vi "get control size.vi"(8 "error in (no error)":errorcluster, 11 "Control in":refnum<class "String Control.lvclass">) -> (0 "error out":errorcluster, 2 "Size":T1, 3 "Control out":refnum<class "String Control.lvclass">)   [LabVIEW 2010, in "String Control.lvclass"]
uses:
  String Control.lvclass
  <vilib>/Utility/miscctls.llb/LVBoundsTypeDef.ctl
  String Control.lvclass/String Control.ctl
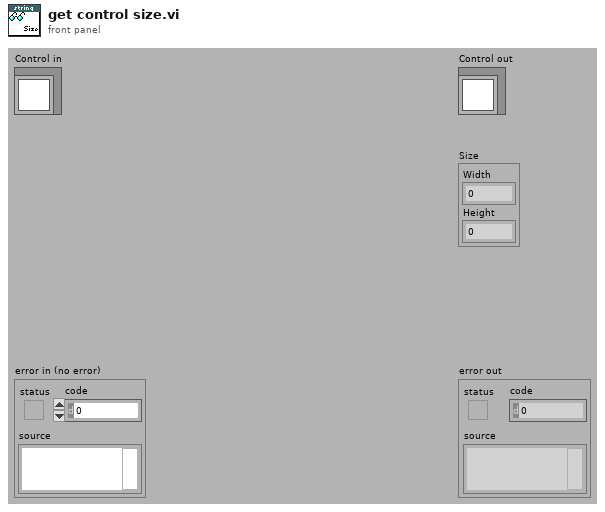
[diagram p1: front panel]
types:
  T1 = typedef "LVBoundsTypeDef.ctl" = cluster{"Width":u32, "Height":u32}
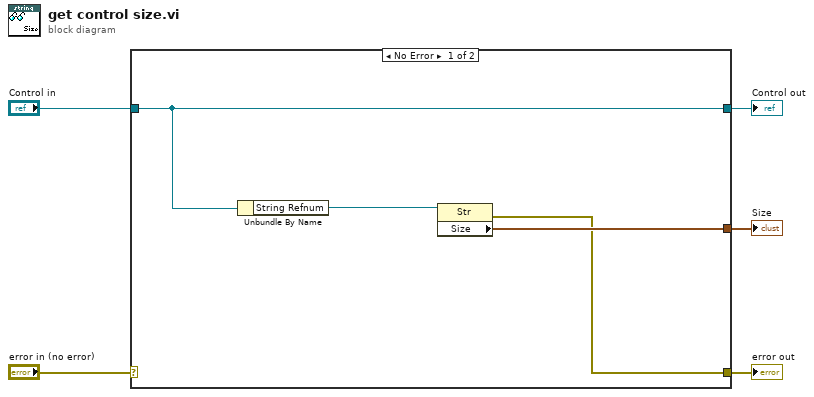
[diagram p0: block diagram]
diagram:
  n1 = case shown="No Error" "error in (no error)" {
    selector: "error in (no error)" -> [_ w11]
    tunnel: [w8 w11] -> w4
    tunnel: [w7 w10] -> w2
    tunnel: "Control in" -> [w7 w10]
    tunnel: [w9 _] -> w1
    frame No Error {
      n2 = Unbundle By Name(w7) -> ("String Refnum"=w6:refnum<vi>)
      n3 = property class="Str"(reference=w6) -> (error out=w8:errorcluster, "Size"=w9:T1)  [unwired: 1 in, 1 out]
    }
    frame Error {
    }
  }
  "error out" <- w4
  "Control out" <- w2
  "Size" <- w1
